vi "FTW-TransferClient-Cancel.vi"(0 "TransferClient.dotNET":refnum<class "FTW-TransferClient-dotNET.lvclass">, 11 "error in":errorcluster) -> (4 "Transfer Client out":refnum<class "FTW-TransferClient-dotNET.lvclass">, 15 "error out":errorcluster)   [LabVIEW 2012, in "FTW-TransferClient-dotNET.lvclass"]
uses:
  FTW-TransferClient-dotNET.lvclass
  FTW-TransferClient.lvclass
  FTW-TransferClient-dotNET.lvclass/FTW-TransferClient-dotNET.ctl
panel:
  # "Inputs"
  # "Outputs"
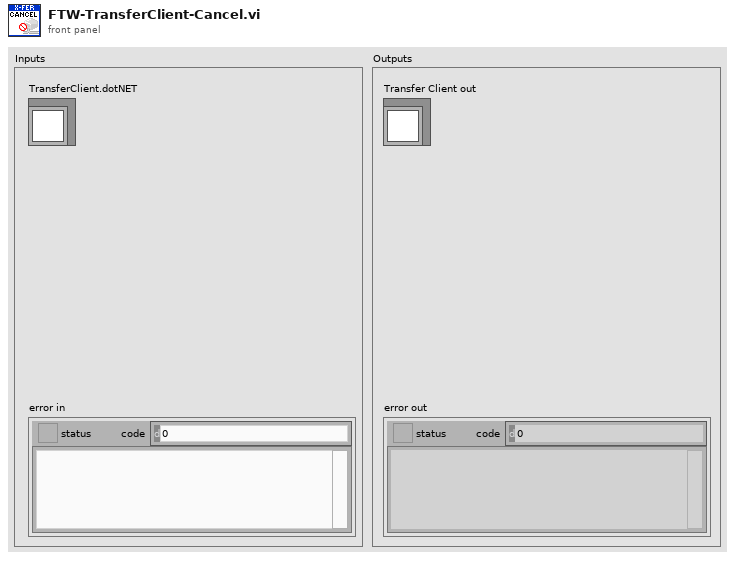
[diagram p1: front panel]
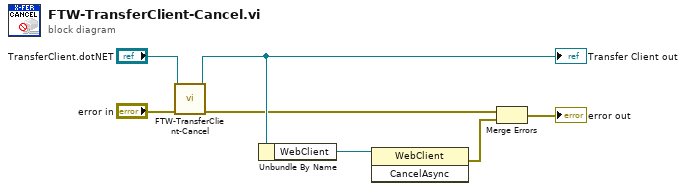
[diagram p0: block diagram]
diagram:
  n1 = call-parent "FTW-TransferClient-Cancel.vi"("Transfer Client"="TransferClient.dotNET", "error in"="error in") -> ("Transfer Client out"=w3:refnum<class "FTW-TransferClient-dotNET.lvclass">, "error out"=w1:errorcluster)  [unwired: 12 in]
  "Transfer Client out" <- w3
  n2 = Unbundle By Name(w3) -> ("WebClient"=w7:refnum<k24>)
  n3 = invoke class="WebClient" method="CancelAsync"(reference=w7) -> (error out=w6:errorcluster)  [unwired: 2 in, 2 out]
  n4 = Merge Errors(w1, w6) -> (→"error out":errorcluster)
